vi "main.vi"() -> ()   [LabVIEW 2011]
panel:
  out "Array":dynamicdata[][](array[waveform])
  out "Multicolumn Listbox":i32(listbox)
  in  "Run Tests":bool
  out "2D Picture":picture
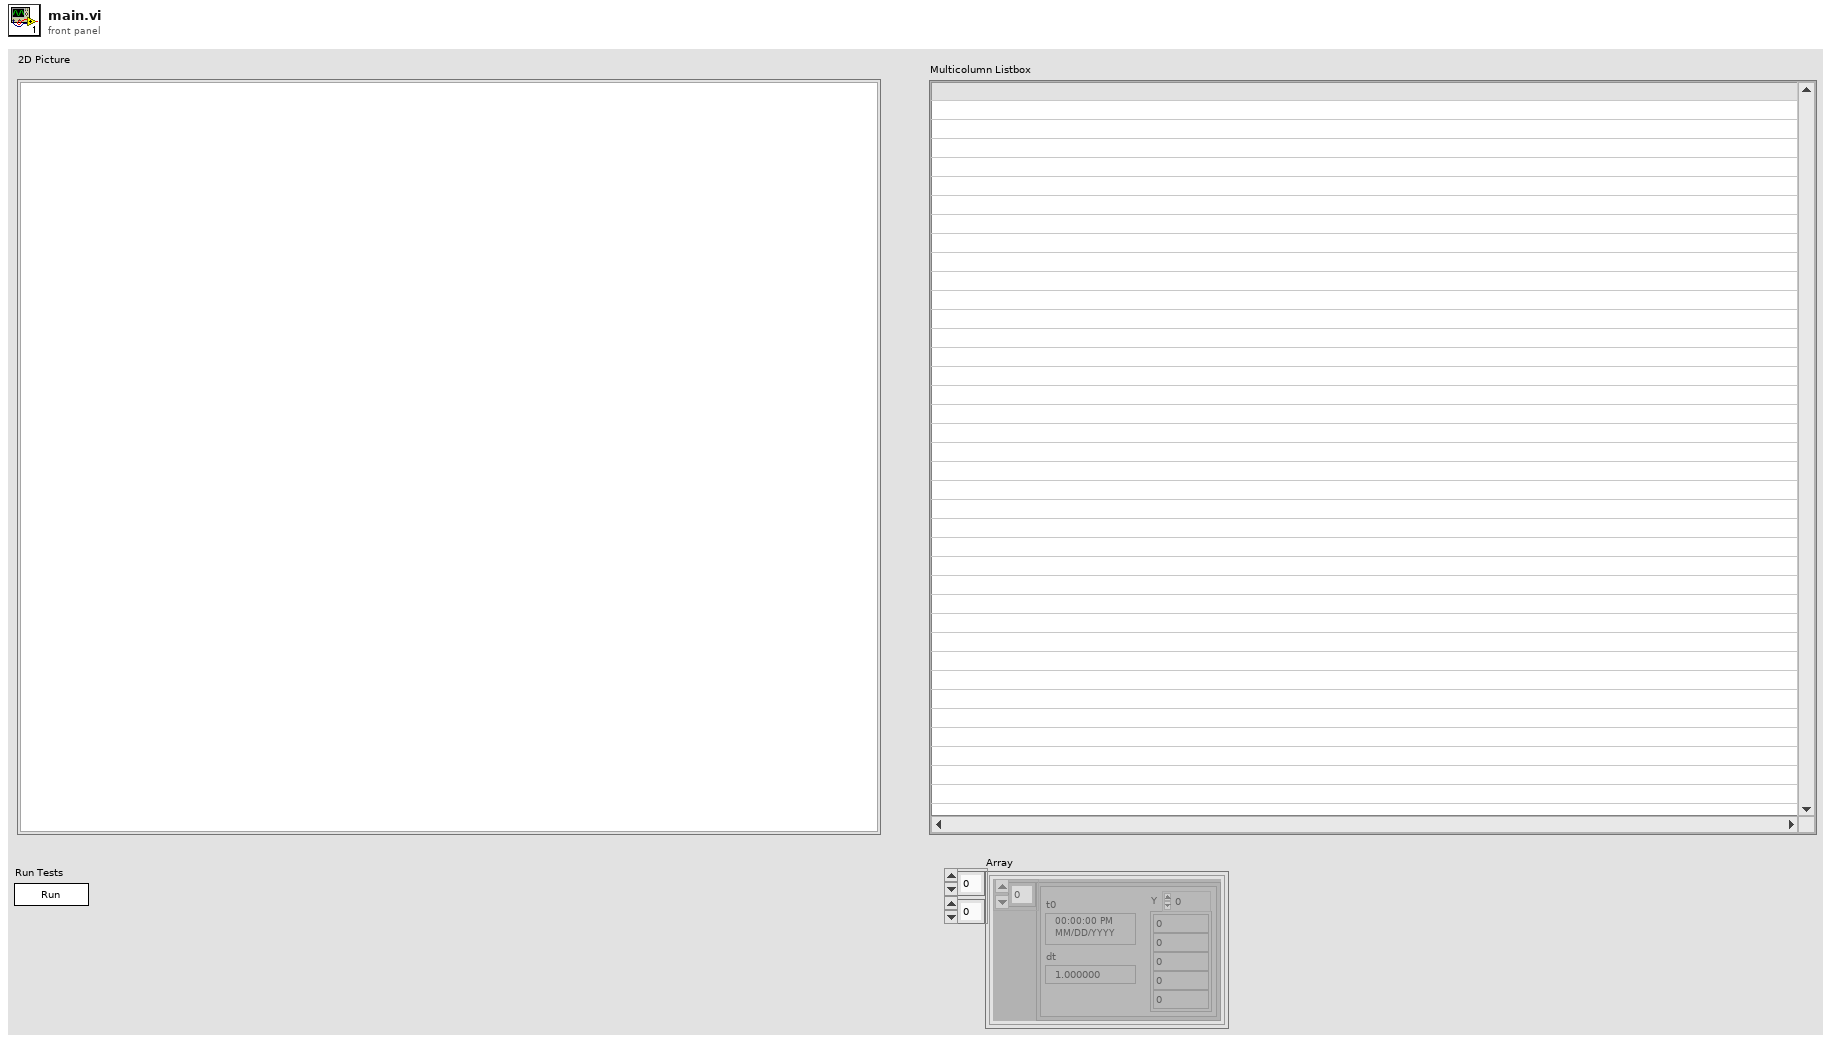
[diagram p1: front panel]
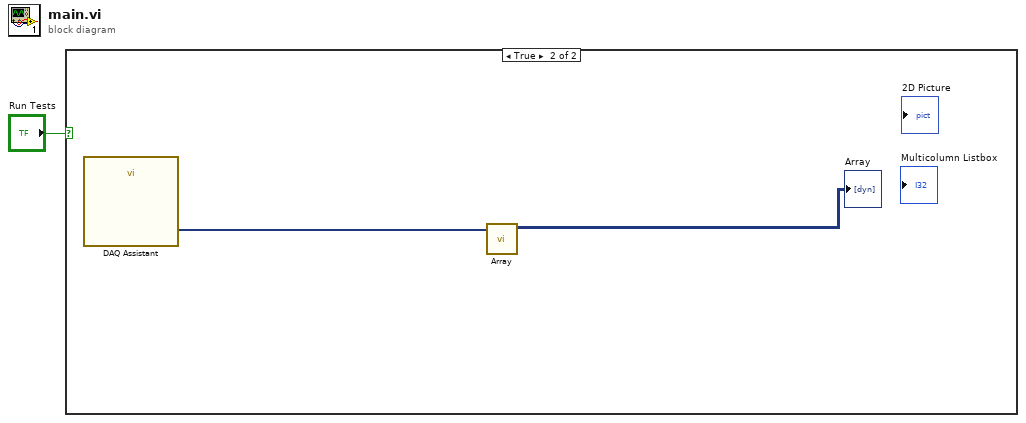
[diagram p0: block diagram]
diagram:
  n1 = case shown="True" "Run Tests" {
    frame False {
    }
    frame True {
      n2 = call "DAQ Assistant"() -> ("data"=w3:dynamicdata)  [unwired: 17 in, 2 out]
      n3 = call "Array.vi"("data"=w3) -> ("Array"=→"Array":dynamicdata[][])  [unwired: 10 in]
    }
  }
